vi "Testing.vi"(11 "VI Refnum in":refnum<vi>) -> (3 "VI Refnum out":refnum<vi>)   [LabVIEW 2010]
uses:
  <vilib>/LabVIEW Icon API/LabVIEW Icon API.lvlib
  <vilib>/LabVIEW Icon API/API_User Layer Data.ctl
  <vilib>/picture/picture.llb/imagedata.ctl
  <vilib>/Utility/miscctls.llb/LVPoint32TypeDef.ctl
  <vilib>/LabVIEW Icon API/lv_icon/Controls/Layer.ctl
  <vilib>/LabVIEW Icon API/lv_icon/classes/Layer/Layer.lvclass
  <vilib>/LabVIEW Icon API/lv_icon/Classes/Icon/Icon.lvclass
  <vilib>/LabVIEW Icon API/lv_icon/Controls/LayerType.ctl
panel:
  in  "error in (no error)":errorcluster
  in  "Color":u32(colorbox)=14446848
  in  "3lettertype":string="DBL"
  out "error out":errorcluster
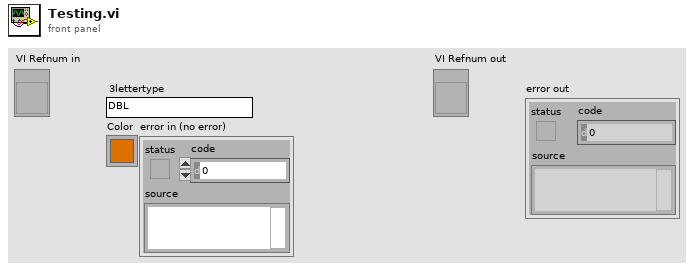
[diagram p1: front panel]
types:
  T1 = cluster{"horizontal":enum16{"left", "center", "right"}, "vertical":enum16{"top", "center", "bottom"}}
  T2 = cluster{"Font Name:":string, "Size":i16, "Strikeout?":bool, "Italic?":bool, "Underline?":bool, "Outline?":bool, "Shadow?":bool, "Bold?":bool}
  T3 = enum16{"User-specified Font", "Application Font", "System Font", "Dialog Font"}
  T4 = typedef "LayerType.ctl" = enum16{"Graphic", "Text", "Tool", "Graphic Drop"}
  T5 = typedef "Layer.ctl" = cluster{"LayerIcon":picture, "LayerName":string, "Opacity":u8, "Visibility?":bool}
  T6 = typedef "LabVIEW Icon API.lvlib/API_User Layer Data.ctl" = cluster{"Layer name":string, "Origin":T7, "Icon image data":T8}
  T7 = typedef "LVPoint32TypeDef.ctl" = cluster{"Horizontal":i32, "Vertical":i32}
  T8 = typedef "imagedata.ctl" = cluster{"image type":i32, "image depth":i32, "image":u8[], "mask":u8[], "colors":u32[], "Rectangle":cluster{"left":i16, "top":i16, "right":i16, "bottom":i16}}
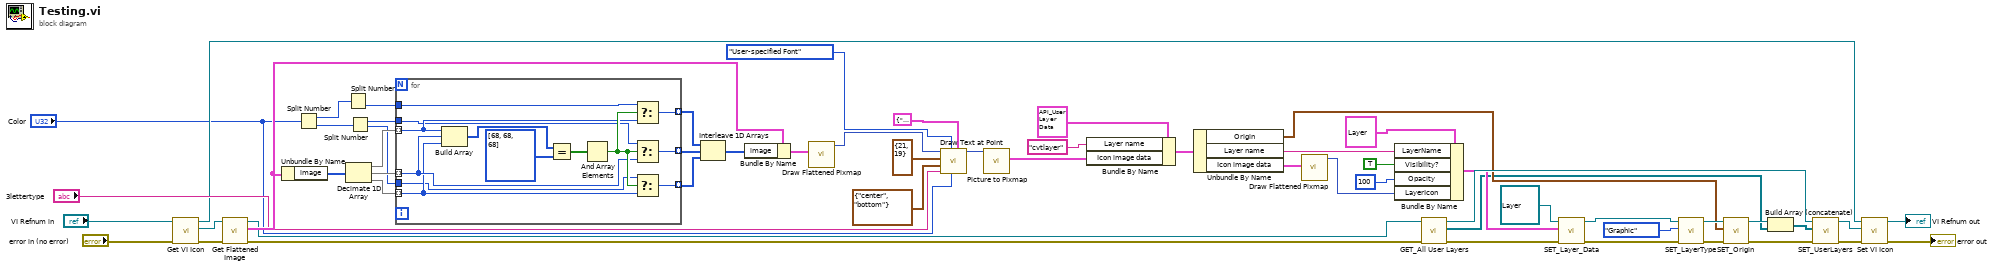
[diagram p0: block diagram]
diagram:
  n1 = call <vilib>:"Get VI Icon.vi"("error in (no error)"="error in (no error)", "VI Refnum in"="VI Refnum in") -> ("error out"=w57:errorcluster, "Icon"=w58:refnum<class "Icon.lvclass">, "VI Refnum out"=w13:refnum<vi>)  [unwired: 7 in]
  n2 = call <vilib>:"Get Flattened Image.vi"("error in (no error)"=w57, "lv_icon.lvlib:Icon.lvclass in"=w58) -> ("error out"=w14:errorcluster, "Color Image"=w44:T8, "lv_icon.lvlib:Icon.lvclass out"=w15:refnum<class "Icon.lvclass">)  [unwired: 6 in, 1 out]
  n3 = Unbundle By Name(w44) -> ("image"=w54:u8[])
  n4 = Split Number(x="Color") -> (hi(x)=w55:u16, lo(x)=w56:u16)
  n5 = Split Number(x=w55) -> (lo(x)=w47:u8)  [unwired: 1 out]
  n6 = Decimate 1D Array(w54) -> (w53:u8[], w52:u8[], w51:u8[])
  n7 = Split Number(x=w56) -> (hi(x)=w46:u8, lo(x)=w45:u8)
  n8 = for {
    tunnel: w53 -> [w67] mode=indexing
    tunnel: w52 -> [w66] mode=indexing
    tunnel: w51 -> [w65] mode=indexing
    tunnel: [w64] -> w50 mode=indexing
    tunnel: [w63] -> w49 mode=indexing
    tunnel: [w62] -> w48 mode=indexing
    tunnel: w47 -> [w61]
    tunnel: w46 -> [w60]
    tunnel: w45 -> [w59]
    n9 = Build Array(w67, w66, w65) -> (w71:u8[])
    n10 = Equal?(x=w71, y=u8[] [68, 68, 68]) -> (x = y?=w69:bool[])
    n11 = And Array Elements(Boolean array=w69) -> (logical AND=w68:bool)
    n12 = Select(t=w61, s=w68, f=w67) -> (s? t:f=w62:u8)
    n13 = Select(t=w60, s=w68, f=w66) -> (s? t:f=w63:u8)
    n14 = Select(t=w59, s=w68, f=w65) -> (s? t:f=w64:u8)
  }
  n15 = Interleave 1D Arrays(w48, w49, w50) -> (w43:u8[])
  n16 = Bundle By Name(cluster=w44, "image"=w43) -> (w42:T8)
  n17 = call <vilib>:"Draw Flattened Pixmap.vi"("image data"=w42) -> ("new picture"=w16:picture)  [unwired: 8 in]
  n18 = call <vilib>:"Draw Text at Point.vi"("[user-specified font]"=T2 {"Font Name:"="Small Fonts", "Size"=9, "Strikeout?"=FALSE, "Italic?"=FALSE, "Underline?"=FALSE, "Outline?"=FALSE, "Shadow?"=FALSE, "Bold?"=FALSE}, "text color(black)"="Color", "desired font(Application)"=T3."User-specified Font", "text"="3lettertype", "alignment(left, top)"=T1 {"horizontal"=enum."center", "vertical"=enum."bottom"}, "origin"=cluster{"x":i16, "y":i16} {"x"=21, "y"=19}, "picture"=w16) -> ("new picture"=w19:picture)  [unwired: 3 in, 1 out]
  n19 = call <vilib>:"Picture to Pixmap.vi"("picture"=w19) -> ("image data"=w40:T8)  [unwired: 9 in, 1 out]
  n20 = Bundle By Name(cluster=T6 {"Layer name"="", "Origin"={"Horizontal"=0, "Vertical"=0}, "Icon image data"={"image type"=0, "image depth"=0, "image"=[], "mask"=[], "colors"=[], "Rectangle"={"left"=0, "top"=0, "right"=0, "bottom"=0}}} ("User layer"), "Layer name"="cvtlayer", "Icon image data"=w40) -> (w20:T6)
  n21 = Unbundle By Name(w20) -> ("Origin"=w24:T7, "Layer name"=w26:string, "Icon image data"=w22:T8)
  n22 = call <vilib>:"Draw Flattened Pixmap.vi"("image data"=w22) -> ("new picture"=w21:picture)  [unwired: 8 in]
  n23 = Bundle By Name(cluster=T5 {"LayerIcon"=bytes[0], "LayerName"="", "Opacity"=0, "Visibility?"=FALSE} ("Data"), "LayerName"=w26, "Visibility?"=TRUE, "Opacity"=u8 100, "LayerIcon"=w21) -> (w29:T5)
  n24 = call-dynamic "GET_All User Layers.vi"("error in (no error)"=w14, "Icon.lvclass in"=w15) -> ("error out"=w34:errorcluster, "User Layer"=w4:refnum<class "Layer.lvclass">[], "Icon.lvclass out"=w35:refnum<class "Icon.lvclass">)  [unwired: 7 in]
  n25 = call-dynamic "SET_Layer_Data.vi"("error in (no error)"=w34, "Data"=w29, "Layer.lvclass in"=refnum<class "Layer.lvclass"> refnum) -> ("error out"=w30:errorcluster, "Layer.lvclass out"=w28:refnum<class "Layer.lvclass">)  [unwired: 1 in, 6 out]
  n26 = call-dynamic "SET_LayerType.vi"("error in (no error)"=w30, "Type"=LayerType."Graphic", "Layer.lvclass in"=w28) -> ("error out"=w23:errorcluster, "Layer.lvclass out"=w25:refnum<class "Layer.lvclass">)  [unwired: 7 out]
  n27 = call-dynamic "SET_Origin.vi"("error in (no error)"=w23, "Point32"=w24, "Layer.lvclass in"=w25) -> ("error out"=w33:errorcluster, "Layer.lvclass out"=w5:refnum<class "Layer.lvclass">)  [unwired: 7 in]
  n28 = Build Array (concatenate)(w5, w4) -> (w36:refnum<class "Layer.lvclass">[])
  n29 = call-dynamic "SET_UserLayers.vi"("error in (no error)"=w33, "Layers"=w36, "Icon.lvclass in"=w35) -> ("error out"=w11:errorcluster, "Icon.lvclass out"=w12:refnum<class "Icon.lvclass">)  [unwired: 7 in]
  n30 = call <vilib>:"Set VI Icon.vi"("error in (no error)"=w11, "Icon"=w12, "VI Refnum in"=w13) -> ("error out"=→"error out":errorcluster, "VI Refnum out"=→"VI Refnum out":refnum<vi>)  [unwired: 7 in]
